vi "Calculate Audio Spectrum.vi"(8 "Error In":errorcluster, 11 "Audio Analyzer In":refnum<class "Audio Analyzer.lvclass">) -> (0 "Error Out":errorcluster, 1 "Invalid Sample Rate":bool, 2 "Audio Spectrum":dbl[](array[numeric]), 3 "Audio Analyzer Out":refnum<class "Audio Analyzer.lvclass">)   [LabVIEW 2021, in "Audio Analyzer.lvclass"]
uses:
  Audio Analyzer.lvclass
  Accessors/FPGA Reference/Get FPGA Reference.vi
  <vilib>/rvi/Analysis/host/Private/Sample Rate To Loop Time (ticks).vi
  <vilib>/Utility/error.llb/Error Cluster From Error Code.vi
  <vilib>/rvi/errors/niLvFpgaAdjustHostInterfaceError.vi
  Public/Controls/FPGA Reference.ctl
  <vilib>/rvi/interface/nirviReadWriteControl/nirviReadWriteControl.xnode
  <vilib>/rvi/interface/nirviMethod/nirviMethod.xnode
  <vilib>/FPGAPlugInAG/Dynamic/niLvFpga_ReadFifo_Dynamic.vi
  <vilib>/rvi/errors/niLvFpgaMergeErrorWithErrorCode.vi
  <vilib>/rvi/Analysis/host/Public/NI_FpgaMspHost.lvlib
  NiFpgaLv.dll
  <vilib>/rvi/interface/Simulation/niFpgaSimulationCallBeginRW.vi
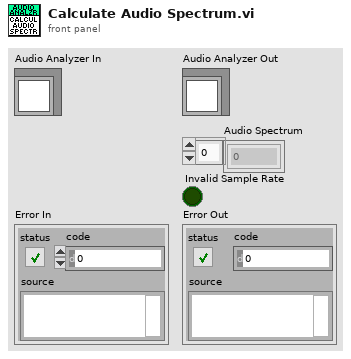
[diagram p1: front panel]
types:
  T1 = typedef "Audio Analyzer.lvclass/FPGA Reference.ctl" = refnum<k20>
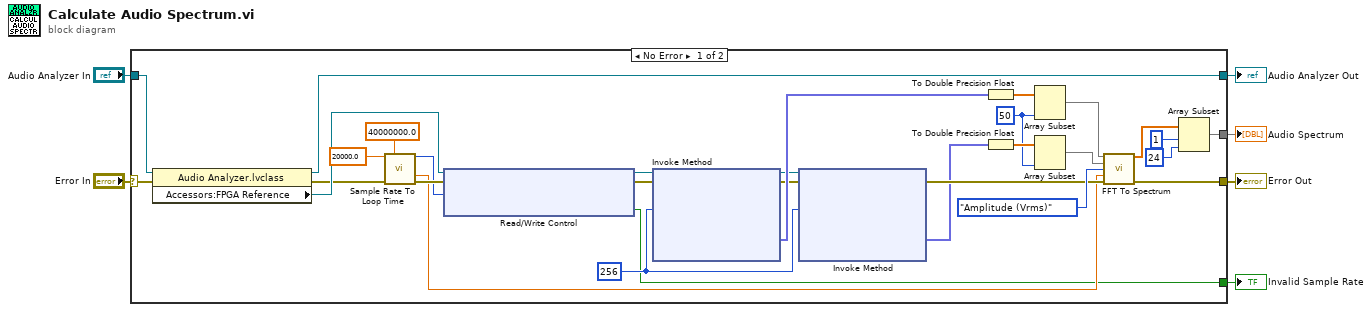
[diagram p0: block diagram]
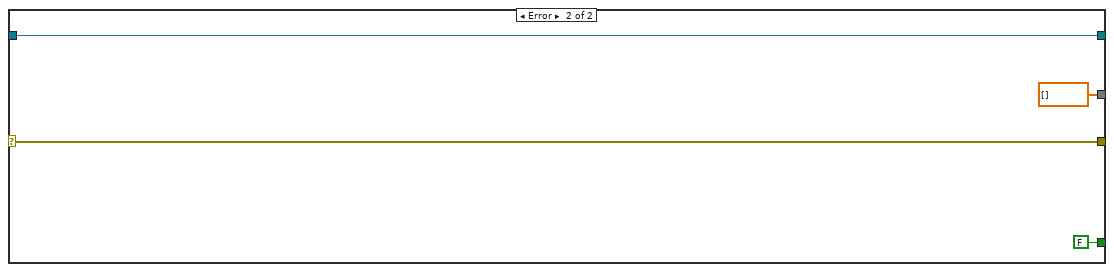
[diagram p2: hidden frame]
diagram:
  n1 = case shown="No Error" "Error In" {
    selector: "Error In" -> [w12 w39]
    tunnel: [w36 w39] -> w6
    tunnel: [w16 FALSE ("Invalid Period")] -> w5
    tunnel: "Audio Analyzer In" -> [w11 w40]
    tunnel: [w8 w40] -> w2
    tunnel: [w7 dbl[] []] -> w1
    frame No Error {
      w31 = 50 ("length")
      w17 = u32 256 ("Number of Elements")
      n2 = property class="Audio Analyzer.lvclass"(reference=w11, error in=w12) -> (reference out=w8:refnum<class "Audio Analyzer.lvclass">, error out=w9:errorcluster, "Accessors:FPGA Reference"=w10:T1)
      n3 = call-poly <vilib>:"Sample Rate To Loop Time.vi"("sample rate (S/s)"=20000.0 ("Sample rate (S/s)"), "FPGA clock rate (Hz)"=40000000.0, "error in (no error)"=w9) -> ("count (ticks/S)"=w21:u32, "actual sample rate (S/s)"=w22:dbl, "error out"=w26:errorcluster)  [unwired: 10 in]
      n4 = xnode "Read/Write Control"("FPGA VI Reference In"=w10, "error in"=w26, "Requested Sample Period (ticks)"=w21) -> ("FPGA VI Reference Out"=w14:T1, "error out"=w19:errorcluster, "Invalid Period"=w16:bool)
      n5 = xnode "Invoke Method"("FPGA VI Reference In"=w14, "error in"=w19, "Number of Elements"=w17) -> ("FPGA VI Reference Out"=w13:T1, "error out"=w18:errorcluster, "Data"=w24:fxp<+/-,25,14>[])  [unwired: 1 in, 1 out]
      n6 = xnode "Invoke Method"("FPGA VI Reference In"=w13, "error in"=w18, "Number of Elements"=w17) -> ("error out"=w25:errorcluster, "Data"=w23:fxp<+/-,25,14>[])  [unwired: 1 in, 2 out]
      n7 = To Double Precision Float(number=w24) -> (double precision float=w30:dbl[])
      n8 = To Double Precision Float(number=w23) -> (double precision float=w32:dbl[])
      n9 = Array Subset(array=w30, length=w31) -> (w33:dbl[])  [unwired: 1 in]
      n10 = Array Subset(array=w32, length=w31) -> (w34:dbl[])  [unwired: 1 in]
      n11 = call <vilib>:"FFT To Spectrum.vi"("real FFT data"=w33, "imaginary FFT data"=w34, "spectrum type"=enum8{"Power (Vrms^2)", "Amplitude (Vrms)"}."Amplitude (Vrms)", "sample rate (S/s)"=w22, "error in (no error)"=w25) -> ("spectrum out"=w27:dbl[], "error out"=w36:errorcluster)  [unwired: 8 in, 1 out]
      n12 = Array Subset(array=w27, index=1, length=24) -> (w7:dbl[])
    }
    frame Error {
    }
  }
  "Invalid Sample Rate" <- w5
  "Error Out" <- w6
  "Audio Analyzer Out" <- w2
  "Audio Spectrum" <- w1
